vi "mat_display_grayscale.vi"() -> ()   [LabVIEW 2015]
uses:
  <vilib>/imath/engines/lvmath2/RunTimeEngine/BuiltInFunctions/view_image/NIMS_view_image.vi
  <vilib>/imathl/engines/lvmath/Functions/Error Handling/Create Error.vi
  <vilib>/imath/engines/lvmath2/RunTimeEngine/ErrorHandling/NIMS_Finalize Error.vi
  <vilib>/picture/picture.llb/Draw 4-Bit Pixmap.vi
panel:
  out "Numeric 2":i32
  out "Numeric":i32
  out "new picture":picture
  out "Array":i32[][](array[numeric])
  out "output 2":i32
  out "output 1":i32
  in  "Path 7":path
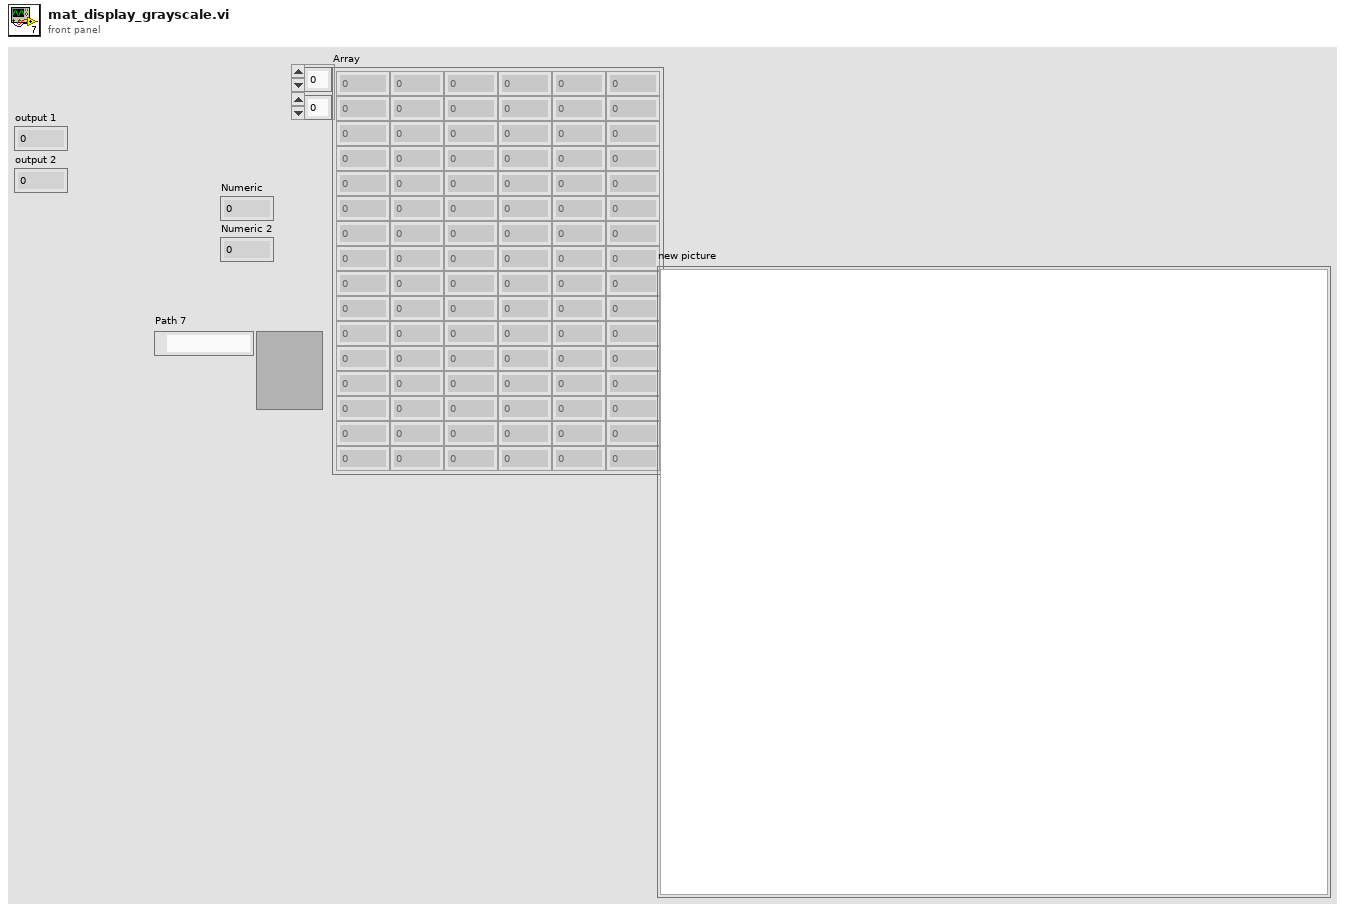
[diagram p1: front panel]
types:
  T1 = enum16{"open", "replace", "create", "open or create", "replace or create", "replace or create with confirmation"}
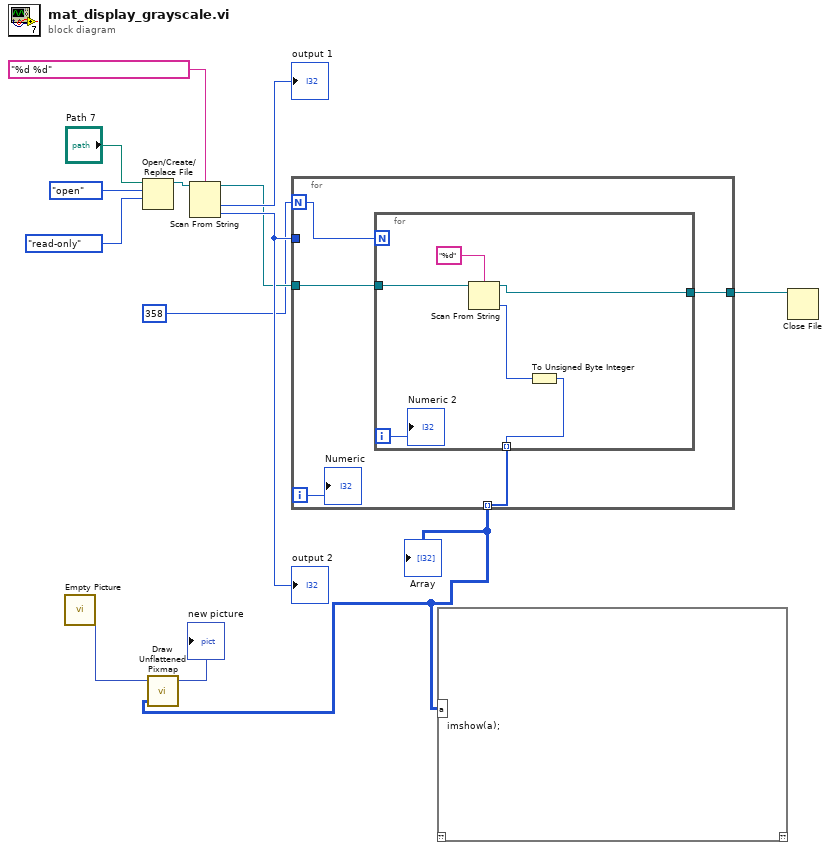
[diagram p0: block diagram]
diagram:
  n1 = call "Empty Picture"() -> ("empty picture"=w4:picture)
  n2 = Open/Create/Replace File(file path (use dialog)="Path 7", operation (0:open)=T1."open", access (0:read/write)=enum16{"read/write", "read-only", "write-only"}."read-only") -> (refnum out=w10:refnum<file>)  [unwired: 3 in, 2 out]
  n3 = Scan From String("%d %d" ("format string"), w10) -> (w6:refnum<file>, output 1=→"output 1":i32, output 2=w7:i32)  [unwired: 3 in, 1 out]
  "output 2" <- w7
  n4 = for {
    N: 358 -> [w14]
    tunnel: w7 -> [_]
    tunnel: w6 -> [w18]
    tunnel: [w17] -> w3 mode=indexing
    tunnel: [w16] -> w5
    i -> [w15]
    n5 = for {
      N: w14 -> [_]
      tunnel: w18 -> [w24]
      tunnel: [w20] -> w17 mode=indexing
      tunnel: [w22] -> w16
      i -> [w19]
      n6 = Scan From String("%d" ("format string"), w24) -> (w22:refnum<file>, output 1=w21:i32)  [unwired: 2 in, 1 out]
      n7 = To Unsigned Byte Integer(number=w21) -> (unsigned 8bit integer=w20:u8)
      "Numeric 2" <- w19
    }
    "Numeric" <- w15
  }
  "Array" <- w3
  n8 = call-poly <vilib>:"Draw Unflattened Pixmap.vi"("picture"=w4, "data"=w3) -> ("new picture"=→"new picture":picture)  [unwired: 7 in]
  n9 = mathscript code="imshow(a);"("a"=w3) -> ()  [unwired: 1 in, 1 out]
  n10 = Close File(refnum=w5) -> ()  [unwired: 1 in, 2 out]
